vi "8.3-Zero Crossing detector test.vi"() -> ()   [LabVIEW 2010]
panel:
  out "Array 2":bool[](array[boolean])
  in  "Array":dbl[](array[numeric])
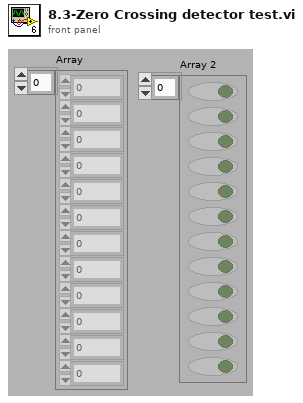
[diagram p1: front panel]
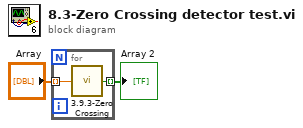
[diagram p0: block diagram]
diagram:
  n1 = for {
    tunnel: "Array" -> [w4] mode=indexing
    tunnel: [w3] -> w1 mode=indexing
    n2 = call "3.9.3-Zero Crossing.vi"("Signal Out"=w4) -> ("Boolean"=w3:bool)
  }
  "Array 2" <- w1
